vi "Test TS Environment Manager - Cache File Creation.vi"() -> (0 "error out":errorcluster)   [LabVIEW 2025]
doc: "Tests creation of the cache file during module startup."
uses:
  <userlib>/_OpenG.lib/file/file.llb/File Exists - Scalar__ogtk.vi
  <vilib>/Utility/config.llb/Read Key (Path).vi
  <userlib>/_OpenG.lib/file/file.llb/openg_file.lvlib
  <vilib>/addons/_JKI Toolkits/Caraya/classes/Test/Test.lvclass
  <vilib>/addons/_JKI Toolkits/Caraya/classes/Assert/Assert.lvclass
  src/Libraries/TS Environment Manager/TS Environment Manager.lvlib
  <vilib>/Utility/config.llb/NI_LVConfig.lvlib
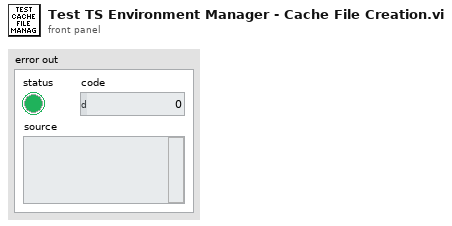
[diagram p1: front panel]
types:
  T1 = typedef "NI_LVConfig.lvlib/Config Data RefNum.ctl" = refnum<k1>
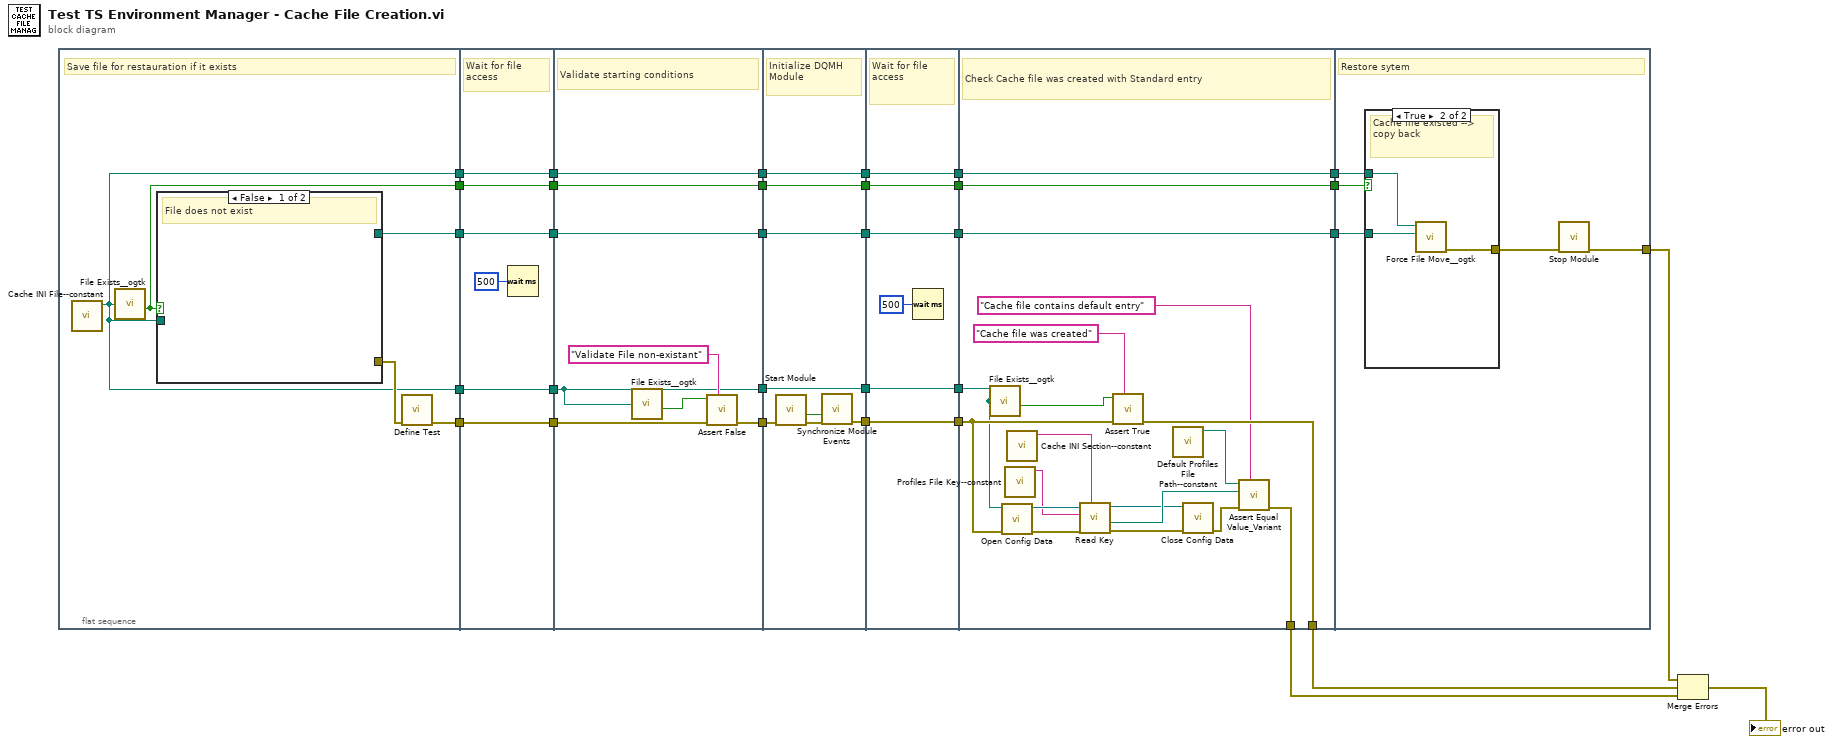
[diagram p0: block diagram]
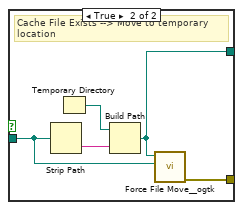
[diagram p2: hidden frame]
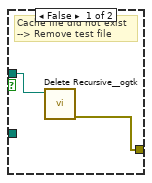
[diagram p3: hidden frame]
diagram:
  n1 = flat-sequence {
    tunnel: [w37] -> w32
    tunnel: [w33] -> w22
    tunnel: [w35] -> w13
    tunnel: [w34] -> w7
    tunnel: [w33] -> w1
    tunnel: w32 -> [w48]
    tunnel: [w48] -> w31
    tunnel: [w46] -> w23
    tunnel: w22 -> [w46]
    tunnel: [w45] -> w14
    tunnel: w13 -> [w45]
    tunnel: [w44] -> w8
    tunnel: w7 -> [w44]
    tunnel: [w43] -> w2
    tunnel: w1 -> [w43]
    tunnel: w31 -> [w56]
    tunnel: w23 -> [w52]
    tunnel: [w55] -> w30
    tunnel: [w52] -> w19
    tunnel: [w51] -> w15
    tunnel: w14 -> [w51]
    tunnel: [w50] -> w9
    tunnel: w8 -> [w50]
    tunnel: [w49] -> w3
    tunnel: w2 -> [w49]
    tunnel: w30 -> [w63]
    tunnel: [w62] -> w29
    tunnel: [w60] -> w20
    tunnel: w19 -> [w60]
    tunnel: [w59] -> w16
    tunnel: w15 -> [w59]
    tunnel: [w58] -> w10
    tunnel: w9 -> [w58]
    tunnel: [w57] -> w4
    tunnel: w3 -> [w57]
    tunnel: w29 -> [w70]
    tunnel: [w70] -> w28
    tunnel: [w68] -> w21
    tunnel: w20 -> [w68]
    tunnel: [w67] -> w17
    tunnel: w16 -> [w67]
    tunnel: [w66] -> w11
    tunnel: w10 -> [w66]
    tunnel: [w65] -> w5
    tunnel: w4 -> [w65]
    tunnel: w28 -> [w89]
    tunnel: w21 -> [w81]
    tunnel: [w85] -> w27
    tunnel: [w84] -> w26
    tunnel: [w73] -> w18
    tunnel: w17 -> [w73]
    tunnel: [w72] -> w12
    tunnel: w11 -> [w72]
    tunnel: [w71] -> w6
    tunnel: w5 -> [w71]
    tunnel: w18 -> [w92]
    tunnel: w12 -> [w91]
    tunnel: w6 -> [w90]
    tunnel: [w93] -> w24
    frame #0 {
      # "Save file for restauration if it exists"
      n2 = call "Cache INI File--constant.vi"() -> ("Cache INI File"=w33:path)  [unwired: 11 in]
      n3 = call-poly <userlib>:"File Exists__ogtk.vi"("file path"=w33) -> ("exists"=w35:bool)  [unwired: 6 in, 1 out]
      n4 = case shown="False" w35 {
        tunnel: w33 -> [_ w39]
        tunnel: [_ w38] -> w34
        tunnel: [_ w42] -> w36
        frame False {
          # "File does not exist"
        }
        frame True {
          # "Cache File Exists --> Move to temporary location"
          n5 = Strip Path(path=w39) -> (name=w40:string)  [unwired: 1 out]
          n6 = Temporary Directory() -> (w41:path)
          n7 = Build Path(base path=w41, name or relative path=w40) -> (appended path=w38:path)
          n8 = call <userlib>:"Force File Move__ogtk.vi"("source"=w39, "target"=w38) -> ("error out"=w42:errorcluster)  [unwired: 4 in, 1 out]
        }
      }
      n9 = call <vilib>:"Define Test.vi"("error in (no error)"=w36) -> ("error out"=w37:errorcluster)  [unwired: 9 in, 1 out]
    }
    frame #1 {
      # "Wait for file access"
      n10 = Wait (ms)(milliseconds to wait=u32 500) -> ()  [unwired: 1 out]
    }
    frame #2 {
      # "Validate starting conditions"
      n11 = call-poly <userlib>:"File Exists__ogtk.vi"("file path"=w52) -> ("exists"=w54:bool)  [unwired: 6 in, 1 out]
      n12 = call <vilib>:"Assert False.vi"("Label"="Validate File non-existant", "error in (no error)"=w56, "False?"=w54) -> ("error out"=w55:errorcluster)  [unwired: 7 in, 1 out]
    }
    frame #3 {
      # "Initialize DQMH Module"
      n13 = call "Start Module.vi"("error in"=w63) -> ("error out"=w64:errorcluster, "Wait for Event Sync?"=w61:bool)  [unwired: 6 in, 3 out]
      n14 = call "Synchronize Module Events.vi"("error in"=w64, "Wait for Event Sync?"=w61) -> ("error out"=w62:errorcluster)  [unwired: 9 in]
    }
    frame #4 {
      # "Wait for file access"
      n15 = Wait (ms)(milliseconds to wait=u32 500) -> ()  [unwired: 1 out]
    }
    frame #5 {
      # "Check Cache file was created with Standard entry"
      n16 = call-poly <userlib>:"File Exists__ogtk.vi"("file path"=w81) -> ("exists"=w82:bool)  [unwired: 6 in, 1 out]
      n17 = call <vilib>:"Open Config Data.vi"("error in (no error)"=w89, "configuration file path"=w81) -> ("error out"=w88:errorcluster, "refnum"=w80:T1)  [unwired: 7 in, 1 out]
      n18 = call "Profiles File Key--constant.vi"() -> ("Profiles File Key"=w78:string)  [unwired: 11 in]
      n19 = call "Cache INI Section--constant.vi"() -> ("Cache INI Section"=w79:string)  [unwired: 11 in]
      n20 = call-poly <vilib>:"Read Key.vi"("section"=w79, "error in (no error)"=w88, "key"=w78, "refnum"=w80) -> ("error out"=w87:errorcluster, "value"=w76:path, "refnum out"=w75:T1)  [unwired: 4 in, 1 out]
      n21 = call <vilib>:"Assert True.vi"("Label"="Cache file was created", "error in (no error)"=w89, "True?"=w82) -> ("error out"=w85:errorcluster)  [unwired: 7 in, 1 out]
      n22 = call "Default Profiles File Path--constant.vi"() -> ("Default Profiles File Path"=w77:path)  [unwired: 11 in]
      n23 = call <vilib>:"Close Config Data.vi"("error in (no error)"=w87, "refnum"=w75) -> ("error out"=w86:errorcluster)  [unwired: 8 in, 1 out]
      n24 = call <vilib>:"Assert Equal Value_Variant.vi"("Label"="Cache file contains default entry", "error in (no error)"=w86, "Actual"=w76, "Expected"=w77) -> ("error out"=w84:errorcluster)  [unwired: 6 in, 1 out]
    }
    frame #6 {
      # "Restore sytem"
      n25 = case shown="True" w92 {
        tunnel: w91 -> [_ w98]
        tunnel: w90 -> [w95 w97]
        tunnel: [w96 w99] -> w94
        frame False {
          # "Cache file did not exist --> Remove test file"
          n26 = call <userlib>:"Delete Recursive__ogtk.vi"("Path"=w95) -> ("error out"=w96:errorcluster)  [unwired: 9 in, 1 out]
        }
        frame True {
          # "Cache file existed --> copy back"
          n27 = call <userlib>:"Force File Move__ogtk.vi"("source"=w98, "target"=w97) -> ("error out"=w99:errorcluster)  [unwired: 4 in, 1 out]
        }
      }
      n28 = call "Stop Module.vi"("error in"=w94) -> ("error out"=w93:errorcluster)  [unwired: 10 in]
    }
  }
  n29 = Merge Errors(w24, w27, w26) -> (→"error out":errorcluster)
